vi "Copy Colors to Screen.vi"(4 "offset y":i32, 6 "offset x":i32, 8 "error in (no error)":errorcluster, 10 "Image":refnum<class "Image.lvclass">, 11 "senseHatDisplay in":refnum<class "RPI.SenseHat.Display.lvclass">) -> (0 "error out":errorcluster, 3 "senseHatDisplay out":refnum<class "RPI.SenseHat.Display.lvclass">)   [LabVIEW 2020, in "RPI.SenseHat.Display.lvlib" / "RPI.SenseHat.Display.lvclass"]
uses:
  RPI.SenseHat.Display.lvclass
  Image/Image.lvclass
  RPI.SenseHat.Display.lvclass/RPI.SenseHat.Display.ctl
panel:
  out "yindex":i32[][](array[numeric])
  out "xindex":i32[](array[numeric])
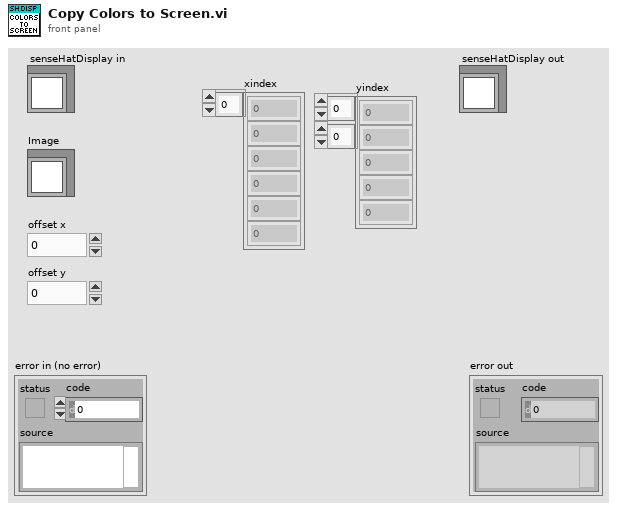
[diagram p1: front panel]
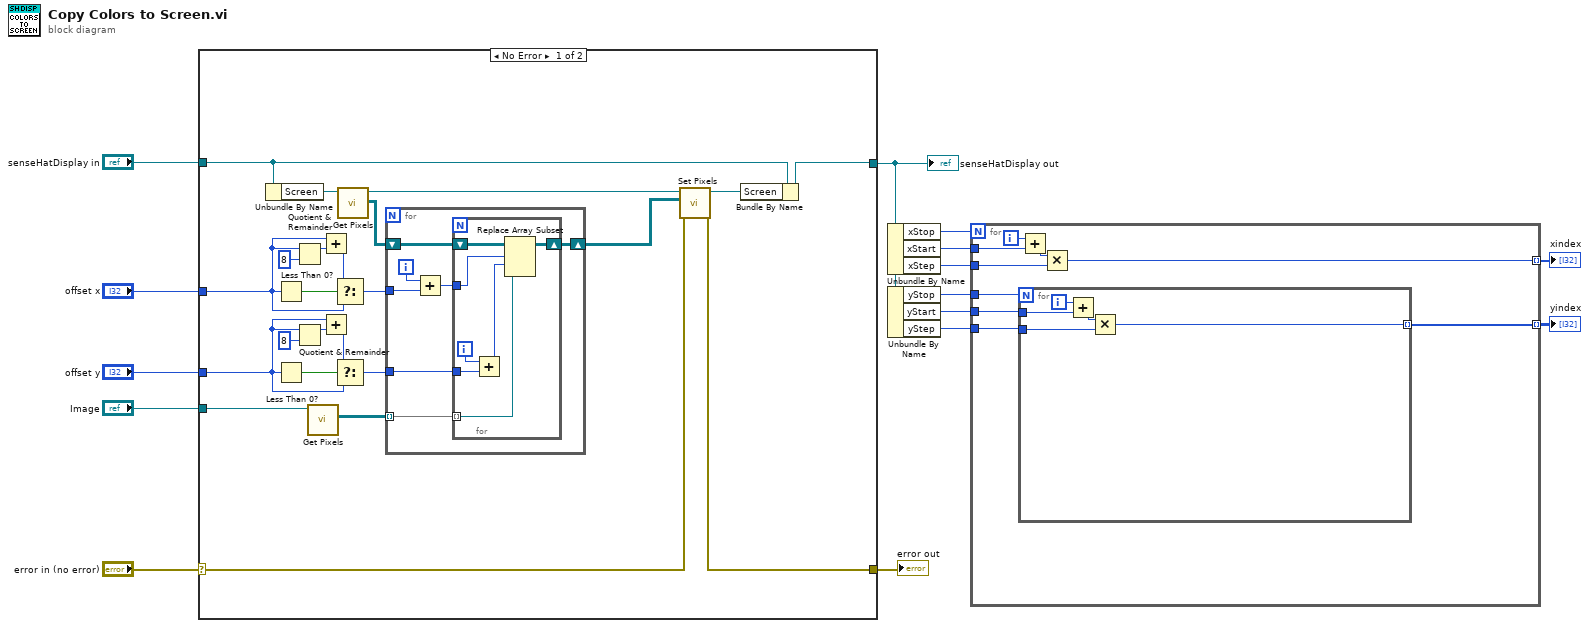
[diagram p0: block diagram]
diagram:
  n1 = case shown="No Error" "error in (no error)" {
    selector: "error in (no error)" -> [w17 w54]
    tunnel: [w16 w54] -> w14
    tunnel: [w28 w53] -> w6
    tunnel: "senseHatDisplay in" -> [w27 w53]
    tunnel: "offset x" -> [w34 _]
    tunnel: "offset y" -> [w29 _]
    tunnel: "Image" -> [w22 _]
    frame No Error {
      n2 = Unbundle By Name(w27) -> ("Screen"=w26:refnum<class "Image.lvclass">)
      n3 = Less Than 0?(x=w34) -> (x < 0?=w38:bool)
      n4 = Less Than 0?(x=w29) -> (x < 0?=w30:bool)
      n5 = Quotient & Remainder(x=w34, y=8) -> (x-y*floor(x/y)=w36:i32)  [unwired: 1 out]
      n6 = Quotient & Remainder(x=w29, y=8) -> (x-y*floor(x/y)=w32:i32)  [unwired: 1 out]
      n7 = call "Get Pixels.vi"("Image in"=w22) -> ("Pixels"=w21:refnum<class "Pixel.lvclass">[][])  [unwired: 8 in, 2 out]
      n8 = Add(x=w34, y=w36) -> (x+y=w35:i32)
      n9 = Add(x=w29, y=w32) -> (x+y=w33:i32)
      n10 = Select(t=w35, s=w38, f=w34) -> (s? t:f=w24:i32)
      n11 = Select(t=w33, s=w30, f=w29) -> (s? t:f=w23:i32)
      n12 = call "Get Pixels.vi"("Image in"=w26) -> ("Pixels"=w25:refnum<class "Pixel.lvclass">[][], "Image out"=w20:refnum<class "Image.lvclass">)  [unwired: 8 in, 1 out]
      n13 = for {
        shift-right: [w44] -> w18
        shift-left: w25 -> [w45]
        tunnel: w24 -> [w42]
        tunnel: w23 -> [w40]
        tunnel: w21 -> [w39] mode=indexing
        i -> [w43]
        n14 = Add(x=w43, y=w42) -> (x+y=w41:i32)
        n15 = for {
          shift-right: [w51] -> w44
          shift-left: w45 -> [w52]
          tunnel: w41 -> [w47]
          tunnel: w40 -> [w50]
          tunnel: w39 -> [w48] mode=indexing
          i -> [w49]
          n16 = Add(x=w49, y=w50) -> (x+y=w46:i32)
          n17 = Replace Array Subset(array=w52, new element=w48, index (row)=w47, index (col)=w46) -> (w51:refnum<class "Pixel.lvclass">[][])
        }
      }
      n18 = call "Set Pixels.vi"("error in (no error)"=w17, "Pixels"=w18, "Image in"=w20) -> ("error out"=w16:errorcluster, "Image out"=w19:refnum<class "Image.lvclass">)  [unwired: 7 in]
      n19 = Bundle By Name(cluster=w27, "Screen"=w19) -> (w28:refnum<class "RPI.SenseHat.Display.lvclass">)
    }
    frame Error {
    }
  }
  "error out" <- w14
  "senseHatDisplay out" <- w6
  n20 = Unbundle By Name(w6) -> ("xStop"=w9:i32, "xStart"=w8:i32, "xStep"=w7:i32)
  n21 = Unbundle By Name(w6) -> ("yStop"=w5:i32, "yStart"=w4:i32, "yStep"=w3:i32)
  n22 = for {
    N: w9 -> [_]
    tunnel: w8 -> [w63]
    tunnel: w7 -> [w60]
    tunnel: w5 -> [w59]
    tunnel: w4 -> [w58]
    tunnel: w3 -> [w57]
    tunnel: [w56] -> w1 mode=indexing
    tunnel: [w55] -> w2 mode=indexing
    i -> [w62]
    n23 = for {
      N: w59 -> [_]
      tunnel: w58 -> [w68]
      tunnel: w57 -> [w65]
      tunnel: [w64] -> w56 mode=indexing
      i -> [w67]
      n24 = Add(x=w67, y=w68) -> (x+y=w66:i32)
      n25 = Multiply(x=w66, y=w65) -> (x*y=w64:i32)
    }
    n26 = Add(x=w62, y=w63) -> (x+y=w61:i32)
    n27 = Multiply(x=w61, y=w60) -> (x*y=w55:i32)
  }
  "xindex" <- w2
  "yindex" <- w1
